vi "Find Midpoint Between Circles.vi"(2 "Circle 1 x and y":cluster{"Pos. X":i32, "Pos. Y":i32}, 3 "Circle 2 x and y":cluster{"Pos. X":i32, "Pos. Y":i32}) -> (0 "Circle 2 dot info":cluster{i32, i32, i32, i32}, 1 "Output circle x and y":cluster{"Pos. X":i32, "Pos. Y":i32})   [LabVIEW 2010]
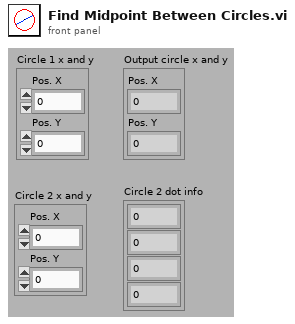
[diagram p1: front panel]
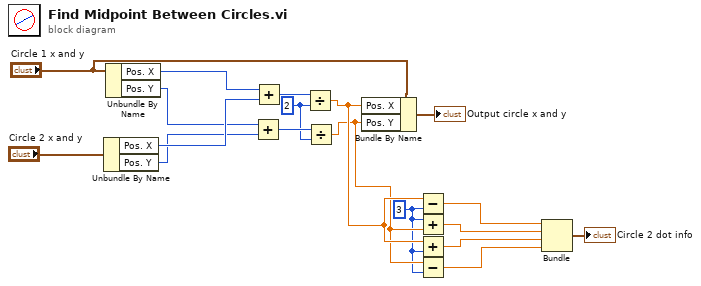
[diagram p0: block diagram]
diagram:
  w1 = 3 ("y")
  w11 = 2 ("y")
  n1 = Unbundle By Name("Circle 2 x and y") -> ("Pos. X"=w16:i32, "Pos. Y"=w14:i32)
  n2 = Unbundle By Name("Circle 1 x and y") -> ("Pos. X"=w17:i32, "Pos. Y"=w15:i32)
  n3 = Add(x=w15, y=w14) -> (x+y=w12:i32)
  n4 = Add(x=w17, y=w16) -> (x+y=w13:i32)
  n5 = Divide(x=w13, y=w11) -> (x/y=w3:dbl)
  n6 = Divide(x=w12, y=w11) -> (x/y=w2:dbl)
  n7 = Bundle By Name(cluster="Circle 1 x and y", "Pos. X"=w3, "Pos. Y"=w2) -> (→"Output circle x and y":cluster{"Pos. X":i32, "Pos. Y":i32})
  n8 = Subtract(x=w3, y=w1) -> (x-y=w8:dbl)
  n9 = Add(x=w1, y=w2) -> (x+y=w7:dbl)
  n10 = Add(x=w3, y=w1) -> (x+y=w6:dbl)
  n11 = Subtract(x=w2, y=w1) -> (x-y=w5:dbl)
  n12 = Bundle(w8, w7, w6, w5) -> (→"Circle 2 dot info":cluster{dbl, dbl, dbl, dbl})  [unwired: 1 in]
